vi "getAnalogValue.vi"(8 "error in (no error)":errorcluster, 11 "ScriptEvent in":refnum<class "ScriptEvent.lvclass">) -> (0 "error out":errorcluster, 2 "analogValue":dbl, 3 "ScriptEvent out":refnum<class "ScriptEvent.lvclass">)   [LabVIEW 2009, in "Tools.lvlib" / "Scripting.lvlib" / "ScriptEvent.lvclass"]
uses:
  ScriptEvent.lvclass
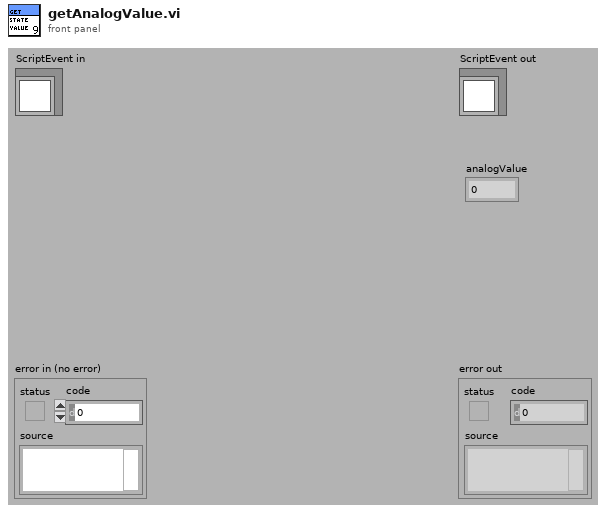
[diagram p1: front panel]
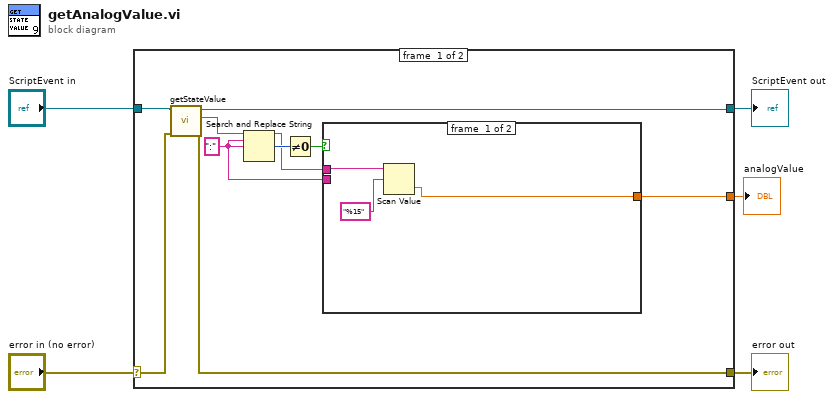
[diagram p0: block diagram]
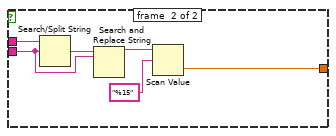
[diagram p2: hidden frame]
diagram:
  n1 = case shown="No Error" "error in (no error)" {
    selector: "error in (no error)" -> [w9 w26]
    tunnel: [w6 w26] -> w4
    tunnel: [w12 w25] -> w2
    tunnel: "ScriptEvent in" -> [w15 w25]
    tunnel: [w7 _] -> w1
    frame #0 {
      w8 = ":"
      n2 = call-dynamic "getStateValue.vi"("error in (no error)"=w9, "ScriptEvent in"=w15) -> ("error out"=w6:errorcluster, "stateValue"=w14:string, "ScriptEvent out"=w12:refnum<class "ScriptEvent.lvclass">)  [unwired: 7 in]
      n3 = Search and Replace String(input string=w14, search string=w8, replace string=w8) -> (result string=w10:string, number of replacements=w13:i32)  [unwired: 5 in, 2 out]
      n4 = Not Equal To 0?(x=w13) -> (x != 0?=w11:bool)
      n5 = case shown="False" w11 {
        tunnel: w10 -> [w17 w24]
        tunnel: w8 -> [_ w22]
        tunnel: [w16 w19] -> w7
        frame #0 {
          n6 = Scan Value(string=w17, format string="%15") -> (value=w16:dbl)  [unwired: 1 in, 1 out]
        }
        frame #1 {
          n7 = Search/Split String(string=w24, search string/char (-)=w22) -> (match + rest of string=w23:string)  [unwired: 1 in, 2 out]
          n8 = Search and Replace String(input string=w23, search string=w22) -> (result string=w21:string)  [unwired: 6 in, 3 out]
          n9 = Scan Value(string=w21, format string="%15") -> (value=w19:dbl)  [unwired: 1 in, 1 out]
        }
      }
    }
    frame #1 {
    }
  }
  "error out" <- w4
  "ScriptEvent out" <- w2
  "analogValue" <- w1
